vi "prepareSelfTerminate.vi"(8 "error in (no error)":errorcluster, 11 "SMO in":refnum<class "SMO.lvclass">) -> (0 "error out":errorcluster, 3 "SMO out":refnum<class "SMO.lvclass">, 4 "SelfTerminate EventReg":refnum<event-registration>)   [LabVIEW 2013, in "SMO.lvclass"]
uses:
  SMO.lvclass
  Typedefs/SMOState --Enum.ctl
  Typedefs/StopProcessEventData--Cluster.ctl
  Typedefs/AbortProcessEventData--Cluster.ctl
  SMO.lvclass/SMO.ctl
  ReftoDVR--SMO.vi
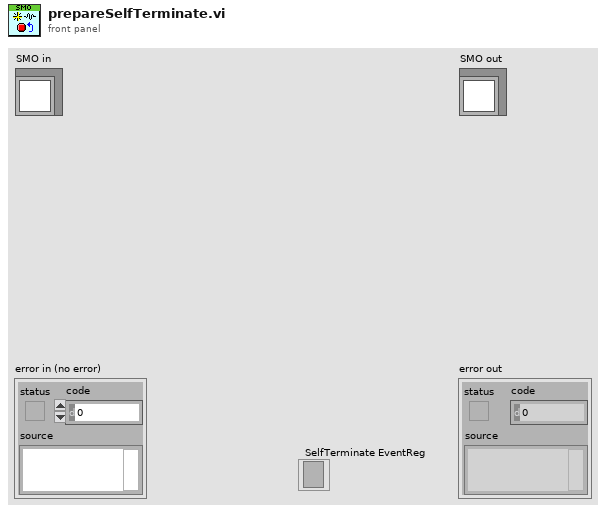
[diagram p1: front panel]
types:
  T1 = typedef "SMO.lvclass/Public Events.ctl" = cluster{"Error":refnum<user-event>, "State":refnum<user-event>, "Reserve State":refnum<user-event>}
  T2 = typedef "SMO.lvclass/Protected Events.ctl" = cluster{"StopProcesses":refnum<user-event>, "AbortProcesses":refnum<user-event>, "Config Changed":refnum<user-event>, "Dependency":refnum<user-event>}
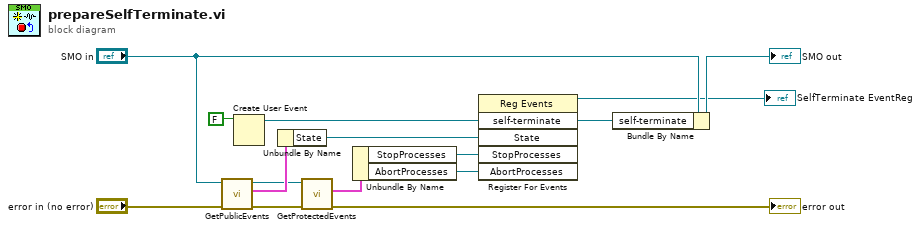
[diagram p0: block diagram]
diagram:
  n1 = call "GetPublicEvents.vi"("error in (no error)"="error in (no error)", "SMO"="SMO in") -> ("error out"=w6:errorcluster, "Public Events"=w9:T1, "SMO out"=w7:refnum<class "SMO.lvclass">)  [unwired: 7 in]
  n2 = Create User Event(user event datatype=FALSE ("self-terminate")) -> (user event=w10:refnum<user-event>)  [unwired: 1 in, 1 out]
  n3 = Unbundle By Name(w9) -> ("State"=w8:refnum<user-event>)
  n4 = call "GetProtectedEvents.vi"("error in (no error)"=w6, "SMO"=w7) -> ("error out"=→"error out":errorcluster, "SMO Protected Events"=w4:T2)  [unwired: 7 in, 1 out]
  n5 = Unbundle By Name(w4) -> ("StopProcesses"=w3:refnum<user-event>, "AbortProcesses"=w2:refnum<user-event>)
  n6 = register-events(w10, w8, w3, w2) -> (reference out=→"SelfTerminate EventReg":refnum<event-registration>)  [unwired: 2 in, 1 out]
  n7 = Bundle By Name(cluster="SMO in", "self-terminate"=w10) -> (→"SMO out":refnum<class "SMO.lvclass">)
